vi "Time for 2.2.vi"() -> ()   [LabVIEW 2013]
panel:
  out "x-y 2":dbl
  out "Numeric 2":dbl
  in  "Numeric":dbl min=0.0 max=30.0 step=1.0
  out "x-y":u32
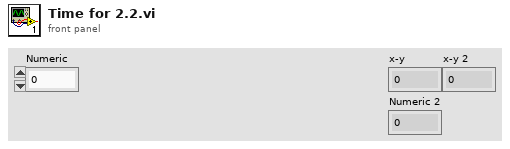
[diagram p1: front panel]
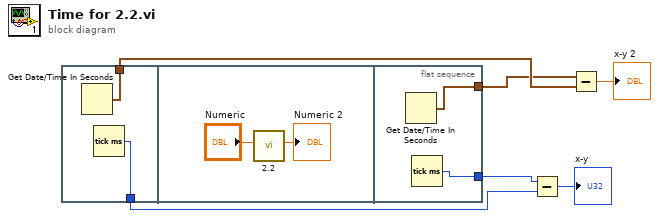
[diagram p0: block diagram]
diagram:
  n1 = flat-sequence {
    tunnel: [w8] -> w6
    tunnel: [w7] -> w2
    tunnel: [w12] -> w5
    tunnel: [w11] -> w1
    frame #0 {
      n2 = Get Date/Time In Seconds() -> (seconds since 1Jan1904=w7:timestamp)
      n3 = Tick Count (ms)() -> (millisecond timer value=w8:u32)
    }
    frame #1 {
      n4 = call "2.2.vi"("Numeric"="Numeric") -> ("Numeric 2"=→"Numeric 2":dbl)  [unwired: 10 in]
    }
    frame #2 {
      n5 = Get Date/Time In Seconds() -> (seconds since 1Jan1904=w11:timestamp)
      n6 = Tick Count (ms)() -> (millisecond timer value=w12:u32)
    }
  }
  n7 = Subtract(x=w5, y=w6) -> (x-y=→"x-y":u32)
  n8 = Subtract(x=w1, y=w2) -> (x-y=→"x-y 2":dbl)
